vi "Display Update During Macro Load.vi"(6 "Macro Error IN":bool, 7 "New Index IN":i32, 8 "error in (no error)":errorcluster, 9 "Macro Array IN":string[](array[string]), 10 "Previous Index IN":i32, 11 "UI control refnums":T1) -> (0 "error out":errorcluster, 3 "New Index OUT":i32, 4 "Macro Error OUT":bool)   [LabVIEW 2012]
doc: "SciScan 1.2 160622"
uses:
  Custom Controls and Typedefs/Macro_MD_UI Control Refnums.ctl
  Custom Controls and Typedefs/Delete Button.ctl
  Custom Controls and Typedefs/Edit Button.ctl
  Custom Controls and Typedefs/Timing Estimate Cluster.ctl
  CommonResource VIs/Timing/Timing Indicator.ctl
  Custom Controls and Typedefs/Load from PSM Button.ctl
  CommonResource VIs/FormatTree&TableStyle_Commands.ctl
  Macro Loop Manager Module/SubVIs/Macro Execution and Timing_Commands.ctl
panel:
  # "(hh:mm:ss)"
  # "(hh:mm:ss)"
  # "(hh:mm:ss)"
  # "(hh:mm:ss)"
  # "(hh:mm:ss)"
  # "(hh:mm:ss)"
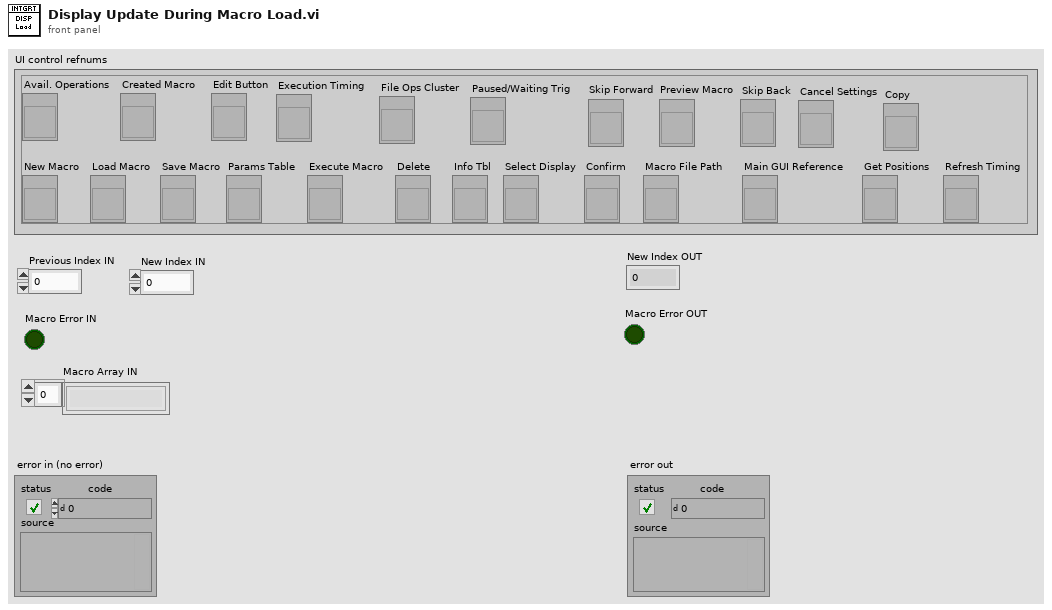
[diagram p1: front panel]
types:
  T1 = typedef "Macro_MD_UI Control Refnums.ctl" = cluster{"Avail. Operations":refnum<vi>, "Created Macro":refnum<vi>, "Load Macro":refnum<vi>, "Save Macro":refnum<vi>, "Params Table":refnum<vi>, "Delete":refnum<vi>, "Edit Button":refnum<vi>, "Execute Macro":refnum<vi>, "Info Tbl":refnum<vi>, "Execution Timing":refnum<vi>, "Select Display":refnum<vi>, "File Ops Cluster":refnum<vi>, "Paused/Waiting Trig":refnum<vi>, "Confirm":refnum<vi>, "New Macro":refnum<vi>, "Preview Macro":refnum<vi>, "Skip Forward":refnum<vi>, "Skip Back":refnum<vi>, "Macro File Path":refnum<vi>, "Main GUI Reference":refnum<vi>, "Cancel Settings":refnum<vi>, "Get Positions":refnum<vi>, "Copy":refnum<vi>, "Refresh Timing":refnum<vi>}
  T2 = typedef "FormatTree&TableStyle_Commands.ctl" = enum16{"Colour Row", "Uncolour Row", "Bold Row", "Unbold Row", "Clear", "UpdateVisibleRows"}
  T3 = typedef "Macro Execution and Timing_Commands.ctl" = enum16{"Initialize (Update FGV & Rst Idx)", "Run", "EstimateTime", "Preview", "Update Macro array (Idx Unchanged)", "Update Index", "Clear Timing Info"}
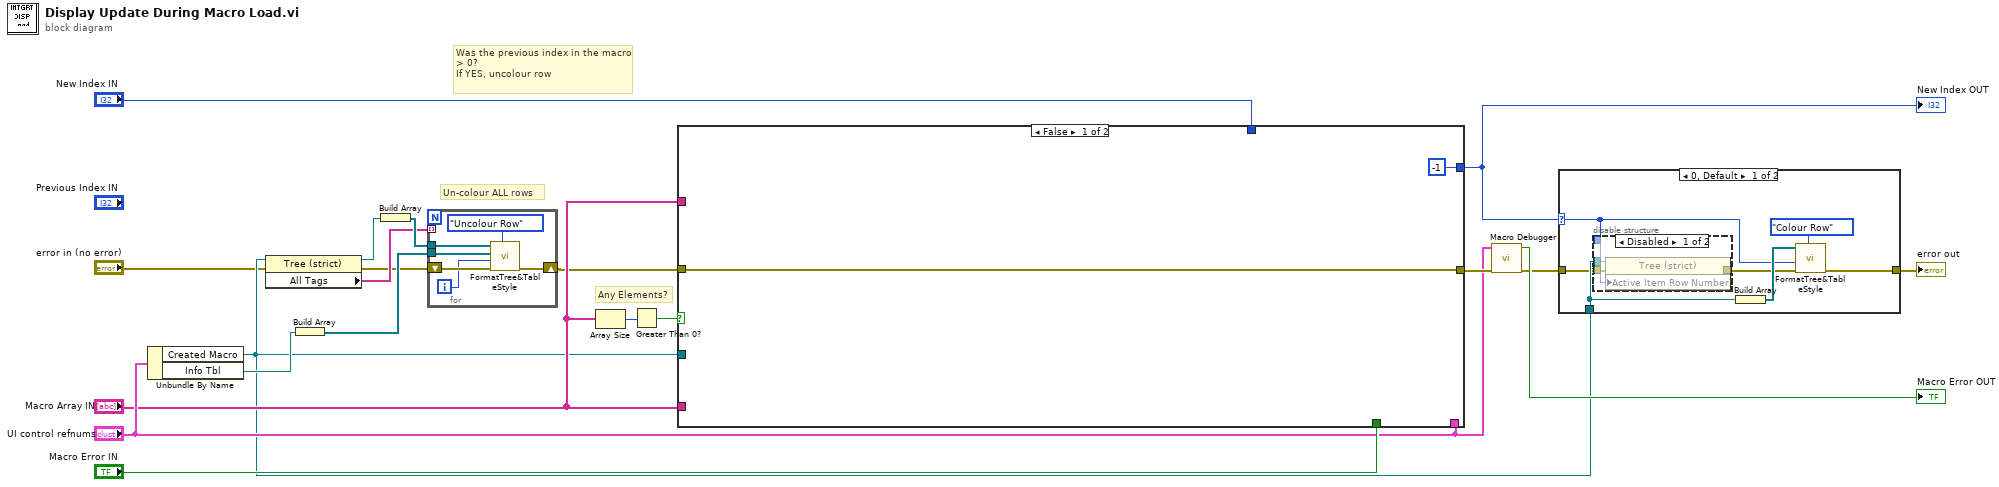
[diagram p0: block diagram]
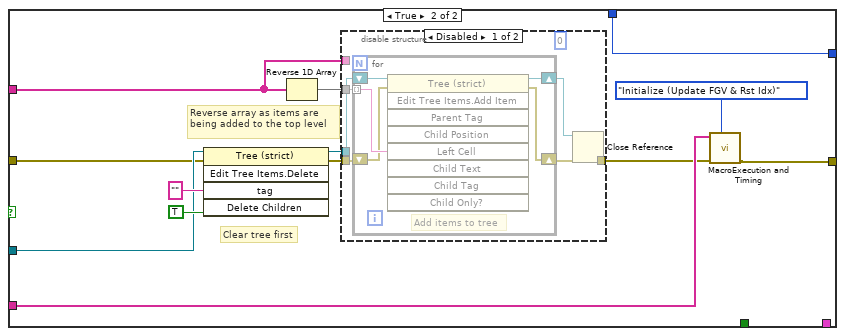
[diagram p4: hidden frame]
diagram:
  # "Un-colour ALL rows"
  # "Any Elements?"
  # "Was the previous index in the macro > 0? \nIf YES, uncolour row"
  n1 = Unbundle By Name("UI control refnums") -> ("Created Macro"=w5:refnum<vi>, "Info Tbl"=w16:refnum<vi>)
  n2 = property class="Tree (strict)"(reference=w5, error in="error in (no error)") -> (reference out=w11:refnum<vi>, error out=w8:errorcluster, "All Tags"=w9:string[])
  n3 = Build Array(w16) -> (w12:refnum<vi>[])
  n4 = Build Array(w11) -> (w10:refnum<vi>[])
  n5 = for {
    tunnel: w12 -> [w24]
    tunnel: w10 -> [w25]
    tunnel: w9 -> [_] mode=indexing
    shift-right: [w21] -> w1
    shift-left: w8 -> [w23]
    i -> [w22]
    n6 = call "FormatTree&TableStyle.vi"("Format Command"=FormatTree&TableStyle_Commands."Uncolour Row", "Error In"=w23, "Row Index"=w22, "Array of Table references"=w24, "Array of Tree references"=w25) -> ("Error Out"=w21:errorcluster)  [unwired: 6 in]
  }
  n7 = Array Size(array="Macro Array IN") -> (size(s)=w18:i32)
  n8 = Greater Than 0?(x=w18) -> (x > 0?=w19:bool)
  n9 = case shown="False" w19 {
    tunnel: w1 -> [w27 w29]
    tunnel: "Macro Array IN" -> [_ w31]
    tunnel: [-1 ("Index") w33] -> w6
    tunnel: w5 -> [_ w36]
    tunnel: [w27 w32] -> w15
    tunnel: "UI control refnums" -> [_ _]
    tunnel: "Macro Array IN" -> [_ w35]
    tunnel: "Macro Error IN" -> [_ _]
    tunnel: "New Index IN" -> [_ w33]
    frame False {
    }
    frame True {
      # "Clear tree first"
      # "Reverse array as items are being added to the top level"
      n10 = invoke class="Tree (strict)" method="Edit Tree Items.Delete"(reference=w36, error in=w29, "tag"="" ("Tag"), "Delete Children"=TRUE ("Delete Children?")) -> (reference out=w37:refnum<vi>, error out=w38:errorcluster)  [unwired: 1 in, 3 out]
      n11 = Reverse 1D Array(array=w31) -> (reversed array=w41:string[])
      n12 = disable-structure shown="Disabled" {
        disable-tunnel: w41 -> [w46 _]
        disable-tunnel: w38 -> [w45 _]
        disable-tunnel: w37 -> [w44 _]
        disable-tunnel: [w43 _] -> w30
        disable-tunnel: w31 -> [_ _]
        frame Disabled {
          (unwired) 0 ("Index")
          n13 = for {
            tunnel: w46 -> [w51] mode=indexing
            shift-right: [w49] -> w47
            shift-left: w45 -> [w50]
            shift-right: [w48] -> w42
            shift-left: w44 -> [w52]
            # "Add items to tree"
            n14 = invoke class="Tree (strict)" method="Edit Tree Items.Add Item"(reference=w52, error in=w50, "Left Cell"=w51) -> (reference out=w48:refnum<vi>, error out=w49:errorcluster)  [unwired: 6 in, 7 out]
          }
          n15 = Close Reference(reference=w42, error in (no error)=w47) -> (error out=w43:errorcluster)
        }
        frame Enabled {
        }
      }
      n16 = call "MacroExecution and Timing.vi"("MacroExecution and Timing Command"=Macro_Execution_and_Timing_Commands."Initialize (Update FGV & Rst Idx)", "Error In"=w30, "Macro IN"=w35) -> ("Error Out"=w32:errorcluster)  [unwired: 3 in, 5 out]
    }
  }
  "New Index OUT" <- w6
  n17 = call "Macro Debugger.vi"("Error In"=w15, "UI control refnums"="UI control refnums") -> ("Error Out"=w4:errorcluster, "Any Error?"=→"Macro Error OUT":bool)  [unwired: 8 in]
  n18 = case shown="0, Default" w6 {
    selector: w6 -> [w54 _]
    tunnel: w5 -> [w57 _]
    tunnel: w4 -> [w55 w64]
    tunnel: [w53 w64] -> w3
    frame 0, Default {
      n19 = disable-structure shown="Disabled" {
        disable-tunnel: w57 -> [w63 _]
        disable-tunnel: [w62 _] -> w56
        disable-tunnel: w55 -> [w61 _]
        disable-tunnel: w54 -> [w60 _]
        frame Disabled {
          n20 = property class="Tree (strict)"(reference=w63, error in=w61, "Active Item Row Number"=w60) -> (error out=w62:errorcluster)  [unwired: 1 out]
        }
        frame Enabled {
        }
      }
      n21 = Build Array(w57) -> (w58:refnum<vi>[])
      n22 = call "FormatTree&TableStyle.vi"("Format Command"=FormatTree&TableStyle_Commands."Colour Row", "Error In"=w56, "Row Index"=w54, "Array of Tree references"=w58) -> ("Error Out"=w53:errorcluster)  [unwired: 7 in]
    }
    frame -1 {
    }
  }
  "error out" <- w3
